vi "Get all Scripts in INI File.vi"(8 "error in (no error)":errorcluster, 11 "configuration file path":path) -> (0 "error out":errorcluster, 1 "All Scipts w/o *":string[](array[string]), 2 "Name of All Scripts":string[](array[string]), 5 "Scripts":cluster{string[]}[](array[cluster]))   [LabVIEW 2018]
uses:
  <vilib>/Utility/config.llb/NI_LVConfig.lvlib
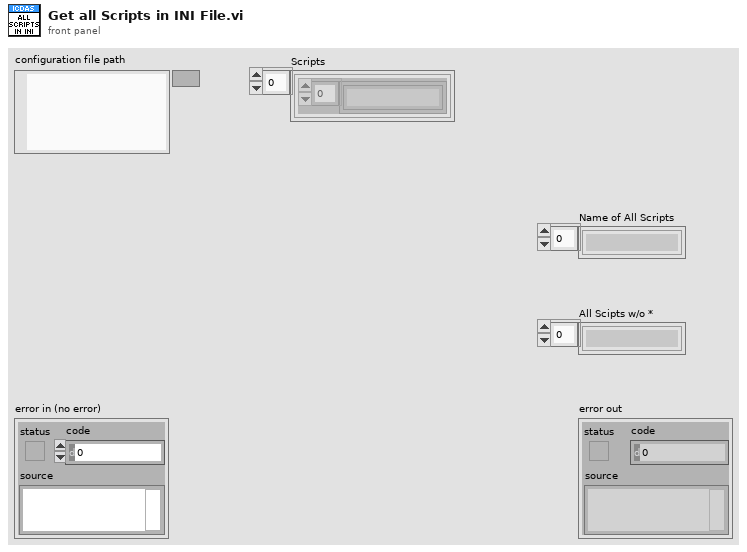
[diagram p1: front panel]
types:
  T1 = typedef "NI_LVConfig.lvlib/Config Data RefNum.ctl" = refnum<k1>
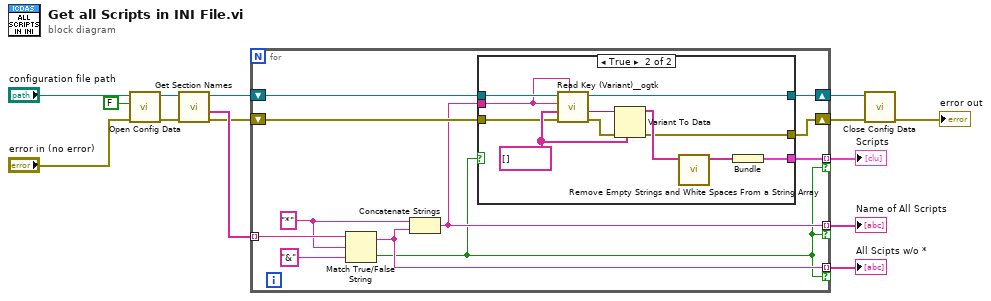
[diagram p0: block diagram]
diagram:
  n1 = call <vilib>:"Open Config Data.vi"("error in (no error)"="error in (no error)", "create file if necessary (T)"=FALSE, "configuration file path"="configuration file path") -> ("error out"=w12:errorcluster, "refnum"=w13:T1)  [unwired: 6 in, 1 out]
  n2 = call <vilib>:"Get Section Names.vi"("error in (no error)"=w12, "refnum"=w13) -> ("error out"=w5:errorcluster, "section names"=w11:string[], "refnum out"=w6:T1)  [unwired: 7 in]
  n3 = for {
    tunnel: w11 -> [w25] mode=indexing
    tunnel: [w17] -> w8 mode=indexing if=w16
    tunnel: [w22] -> w7 mode=indexing if=w16
    shift-right: [w20] -> w4
    shift-left: w6 -> [w21]
    shift-right: [w18] -> w2
    shift-left: w5 -> [w19]
    tunnel: [w15] -> w1 mode=indexing if=w16
    w23 = "*" ("true string")
    n4 = Match True/False String(2:"&" ("false string"), 3:w23, 4:w25) -> (0:w16:bool, 1:w22:string)
    n5 = Concatenate Strings(w23, w22) -> (w17:string)
    n6 = case shown="True" w16 {
      tunnel: w21 -> [w27 w35]
      tunnel: [w27 w34] -> w20
      tunnel: w19 -> [w26 w33]
      tunnel: [w26 w30] -> w18
      tunnel: w17 -> [_ w32]
      tunnel: [_ w29] -> w15
      frame False {
      }
      frame True {
        w37 = string[] []
        n7 = call <userlib>:"Read Key (Variant)__ogtk.vi"("section"=w32, "error in (no error)"=w33, "type"=w37, "key (optional)"=w32, "refnum"=w35) -> ("error out"=w36:errorcluster, "key-value"=w38:variant, "refnum out"=w34:T1)  [unwired: 3 in, 1 out]
        n8 = Variant To Data(error in=w36, type=w37, Variant=w38) -> (data=w31:string[], error out=w30:errorcluster)
        n9 = call "Remove Empty Strings and White Spaces From a String Array.vi"("Array in"=w31) -> ("Array out"=w28:string[])  [unwired: 10 in]
        n10 = Bundle("Array out"=w28) -> (w29:cluster{"Array out":string[]})  [unwired: 1 in]
      }
    }
  }
  "Name of All Scripts" <- w8
  "All Scipts w/o *" <- w7
  "Scripts" <- w1
  n11 = call <vilib>:"Close Config Data.vi"("error in (no error)"=w2, "refnum"=w4) -> ("error out"=→"error out":errorcluster)  [unwired: 8 in, 1 out]
